vi "7_seg_cluster_disp__7_3.vi"() -> ()   [LabVIEW 2026]
panel:
  in  "Array":cluster{}[](array[cluster])
  in  "Combo Box":string(combo)
  out "output cluster":T1
  in  "2":bool
  in  "op":T2
  out "x > y?":bool[](array[boolean])
  in  "Cluster 2":cluster{"Array":dbl[]}
  in  "Cluster":cluster{"Array":dbl[]}
  # "7 segment display"
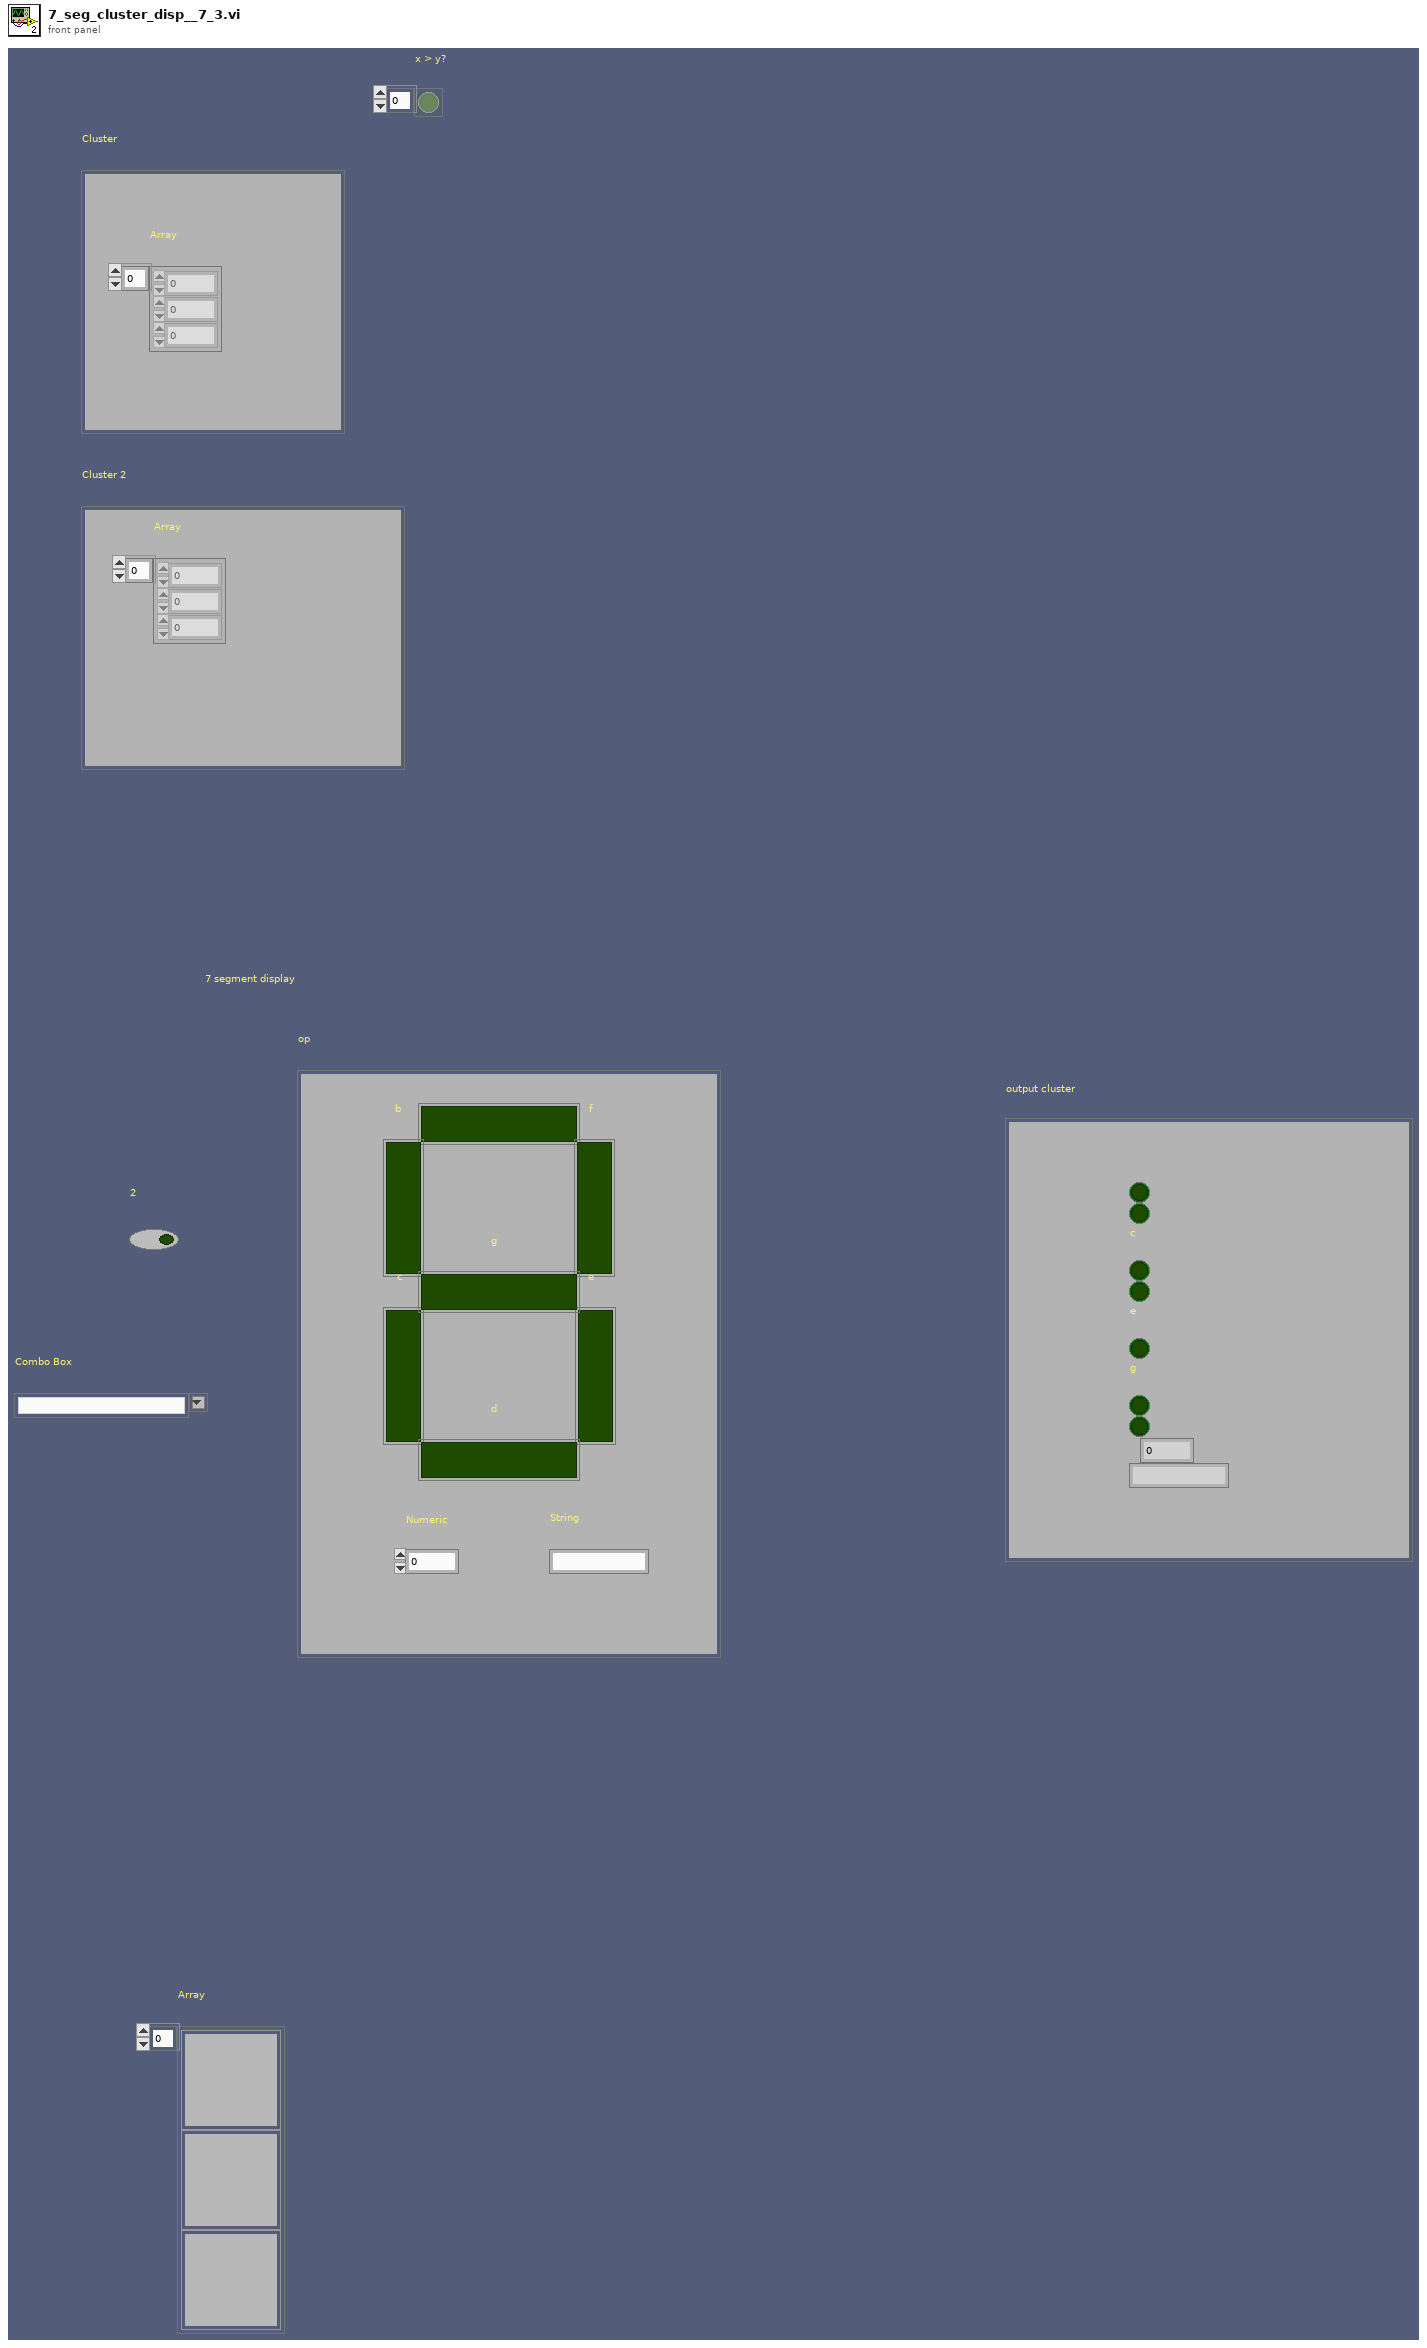
[diagram p1: front panel]
types:
  T1 = cluster{bool, bool, "c":bool, bool, "e":bool, "g":bool, bool, dbl, string}
  T2 = cluster{"a":bool, "b":bool, "c":bool, "f":bool, "e":bool, "g":bool, "d":bool, "Numeric":dbl, "String":string}
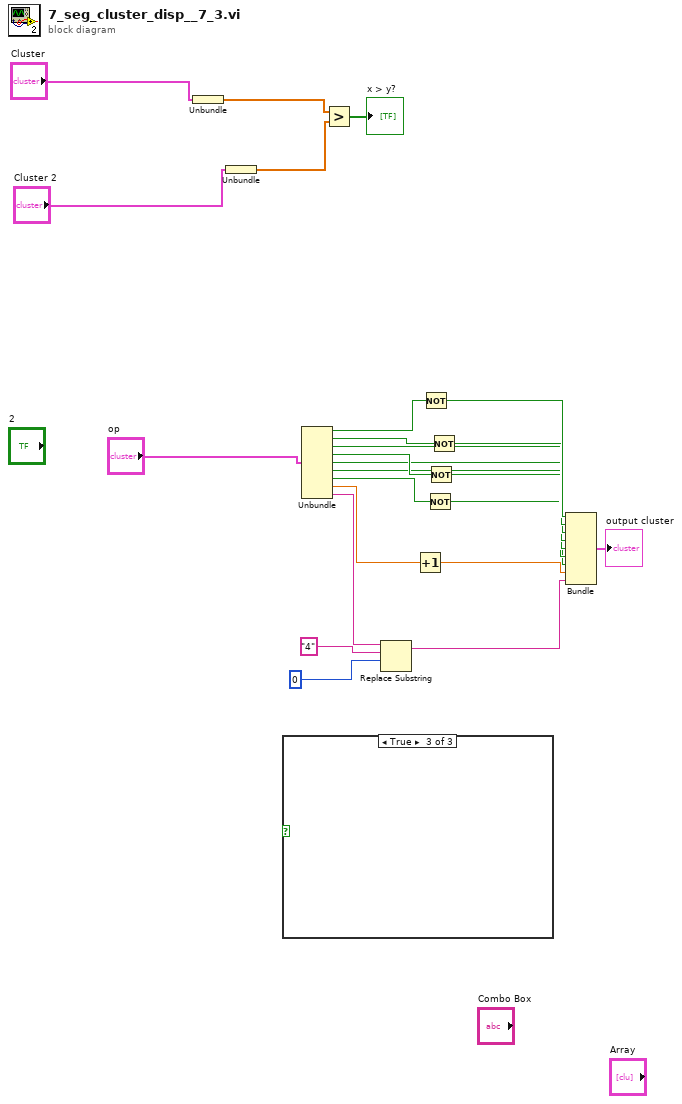
[diagram p0: block diagram]
diagram:
  n1 = Unbundle("Cluster") -> ("Array"=w21:dbl[])
  n2 = Unbundle("Cluster 2") -> ("Array"=w22:dbl[])
  n3 = case shown="True" {
    selector: _ -> [_ _ _]
    frame False {
    }
    frame Default {
    }
    frame True {
    }
  }
  n4 = Unbundle("op") -> ("a"=w17:bool, "b"=w18:bool, "c"=w8:bool, "f"=w16:bool, "e"=w6:bool, "g"=w5:bool, "d"=w15:bool, "Numeric"=w14:dbl, "String"=w13:string)
  n5 = Greater?(x=w21, y=w22) -> (0:→"x > y?":bool[])
  n6 = Replace Substring(3:0, 4:"4", 5:w13) -> (1:w2:string)  [unwired: 1 in, 1 out]
  n7 = Increment(x=w14) -> (x+1=w3:dbl)
  n8 = Not(x=w17) -> (.not. x?=w10:bool)
  n9 = Not(x=w15) -> (.not. x?=w4:bool)
  n10 = Not(x=w16) -> (.not. x?=w7:bool)
  n11 = Not(x=w18) -> (.not. x?=w9:bool)
  n12 = Bundle(w10, w9, "c"=w8, w7, "e"=w6, "g"=w5, w4, w3, w2) -> (→"output cluster":T1)  [unwired: 1 in]
